vi "LEP_RV_UVSetMicroLib.vi"(7 "Use MicroLib":bool, 8 "error in (no error)":errorcluster, 11 "uVision Project":path) -> (0 "error out":errorcluster)   [LabVIEW 2011]
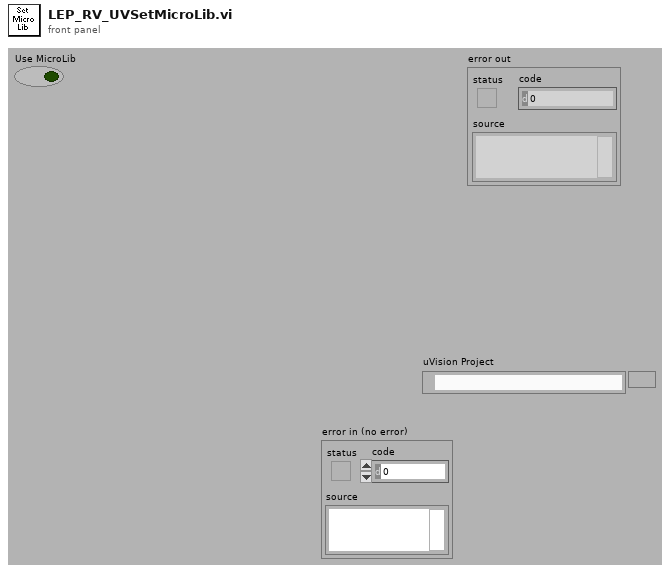
[diagram p1: front panel]
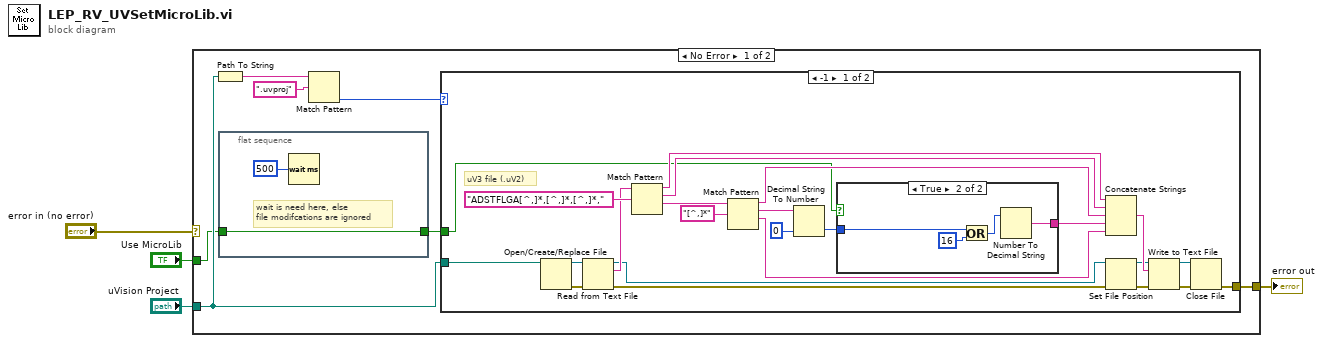
[diagram p0: block diagram]
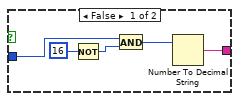
[diagram p2: hidden frame]
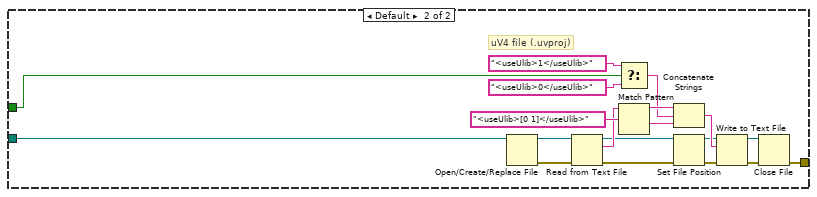
[diagram p3: hidden frame]
diagram:
  n1 = case shown="No Error" "error in (no error)" {
    selector: "error in (no error)" -> [_ w66]
    tunnel: [w7 w66] -> w3
    tunnel: "uVision Project" -> [w8 _]
    tunnel: "Use MicroLib" -> [w6 _]
    frame No Error {
      n2 = Path To String(path=w8) -> (string=w11:string)
      n3 = flat-sequence {
        tunnel: w6 -> [w12]
        tunnel: [w12] -> w5
        frame #0 {
          # "wait is need here, else\nfile modifcations are ignored"
          n4 = Wait (ms)(milliseconds to wait=u32 500) -> ()  [unwired: 1 out]
        }
      }
      n5 = Match Pattern(string=w11, regular expression=".uvproj") -> (offset past match=w9:i32)  [unwired: 1 in, 3 out]
      n6 = case shown="-1" w9 {
        tunnel: w8 -> [w29 w58]
        tunnel: w5 -> [w16 w62]
        tunnel: [w28 w47] -> w7
        frame -1 {
          # "uV3 file (.uV2)"
          n7 = Open/Create/Replace File(file path (use dialog)=w29) -> (refnum out=w36:refnum<file>, error out=w35:errorcluster)  [unwired: 5 in, 1 out]
          n8 = Read from Text File(file (use dialog)=w36, error in=w35) -> (refnum out=w33:refnum<file>, text=w34:string, error out=w32:errorcluster)  [unwired: 2 in, 1 out]
          n9 = Match Pattern(string=w34, regular expression="ADSTFLGA[^,]*,[^,]*,[^,]*,") -> (before substring=w25:string, match substring=w24:string, after substring=w27:string)  [unwired: 1 in, 1 out]
          n10 = Match Pattern(string=w27, regular expression="[^,]*") -> (before substring=w23:string, match substring=w18:string, after substring=w22:string)  [unwired: 1 in, 1 out]
          n11 = Decimal String To Number(string=w18, default (0L)=u32 0 ("default (0 I32)")) -> (number=w17:u32)  [unwired: 1 in, 1 out]
          n12 = case shown="True" w16 {
            tunnel: w17 -> [w41 w46]
            tunnel: [w40 w44] -> w15
            frame False {
              n13 = Not(x=u32 16) -> (.not. x?=w38:u32)
              n14 = And(x=w41, y=w38) -> (x .and. y?=w42:u32)
              n15 = Number To Decimal String(number=w42) -> (decimal integer string=w40:string)  [unwired: 1 in]
            }
            frame True {
              n16 = Or(x=w46, y=u32 16) -> (x .or. y?=w45:u32)
              n17 = Number To Decimal String(number=w45) -> (decimal integer string=w44:string)  [unwired: 1 in]
            }
          }
          n18 = Concatenate Strings(w25, w24, w23, w15, w22) -> (w21:string)
          n19 = Set File Position(refnum=w33, error in=w32) -> (refnum out=w20:refnum<file>, error out=w19:errorcluster)  [unwired: 2 in]
          n20 = Write to Text File(file (use dialog)=w20, text=w21, error in=w19) -> (refnum out=w31:refnum<file>, error out=w30:errorcluster)  [unwired: 1 in, 1 out]
          n21 = Close File(refnum=w31, error in=w30) -> (error out=w28:errorcluster)  [unwired: 1 out]
        }
        frame Default {
          # "uV4 file (.uvproj)"
          n22 = Open/Create/Replace File(file path (use dialog)=w58) -> (refnum out=w57:refnum<file>, error out=w56:errorcluster)  [unwired: 5 in, 1 out]
          n23 = Read from Text File(file (use dialog)=w57, error in=w56) -> (refnum out=w53:refnum<file>, text=w55:string, error out=w51:errorcluster)  [unwired: 2 in, 1 out]
          n24 = Select(t="<useUlib>1</useUlib>", s=w62, f="<useUlib>0</useUlib>") -> (s? t:f=w59:string)
          n25 = Match Pattern(string=w55, regular expression="<useUlib>[0 1]</useUlib>") -> (before substring=w64:string, after substring=w63:string)  [unwired: 1 in, 2 out]
          n26 = Concatenate Strings(w64, w59, w63) -> (w54:string)
          n27 = Set File Position(refnum=w53, error in=w51) -> (refnum out=w52:refnum<file>, error out=w50:errorcluster)  [unwired: 2 in]
          n28 = Write to Text File(file (use dialog)=w52, text=w54, error in=w50) -> (refnum out=w49:refnum<file>, error out=w48:errorcluster)  [unwired: 1 in, 1 out]
          n29 = Close File(refnum=w49, error in=w48) -> (error out=w47:errorcluster)  [unwired: 1 out]
        }
      }
    }
    frame Error {
    }
  }
  "error out" <- w3
